vi "FlatToRichnixnet_grpc_ConvertTimestamp100nsTo1nsResponse.vi"(5 "OutputClusterType":T1, 11 "InputCluster":T2) -> (3 "OutputCluster":T1)   [LabVIEW 2025, in "grpc-xnet_client.lvlib"]
uses:
  grpc-xnet_client.lvlib
  nixnet_grpc_ConvertTimestamp100nsTo1nsResponse_Flat.ctl
  nixnet_grpc_ConvertTimestamp100nsTo1nsResponse.ctl
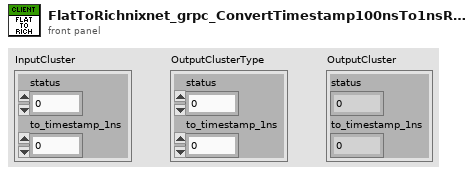
[diagram p1: front panel]
types:
  T1 = typedef "grpc-xnet_client.lvlib/nixnet_grpc_ConvertTimestamp100nsTo1nsResponse.ctl" = cluster{"status":i32, "to_timestamp_1ns":u64}
  T2 = typedef "grpc-xnet_client.lvlib/nixnet_grpc_ConvertTimestamp100nsTo1nsResponse_Flat.ctl" = cluster{"status":i32, "to_timestamp_1ns":u64}
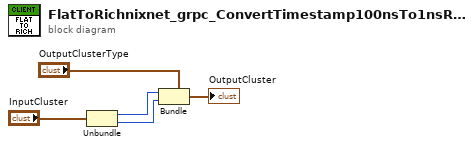
[diagram p0: block diagram]
diagram:
  n1 = Unbundle "Unbundle"("InputCluster") -> ("status"=w2:i32, "to_timestamp_1ns"=w1:u64)
  n2 = Bundle "Bundle"(cluster="OutputClusterType", "status"=w2, "to_timestamp_1ns"=w1) -> (→"OutputCluster":T1)
